vi "Lesson3 - Implicit Property Node demo.vi"() -> ()   [LabVIEW 2013]
panel:
  in  "Stop Button 2":bool
  out "Tank 2":dbl(slide) scale=0.0..10.0
  in  "Vertical Fill Slide 2":dbl(slide) scale=0.0..10.0
  in  "Vertical Fill Slide":dbl(slide) scale=0.0..10.0
  out "Tank":dbl(slide) scale=0.0..10.0
  in  "Stop Button":bool
  # "this is Property Node demonstration"
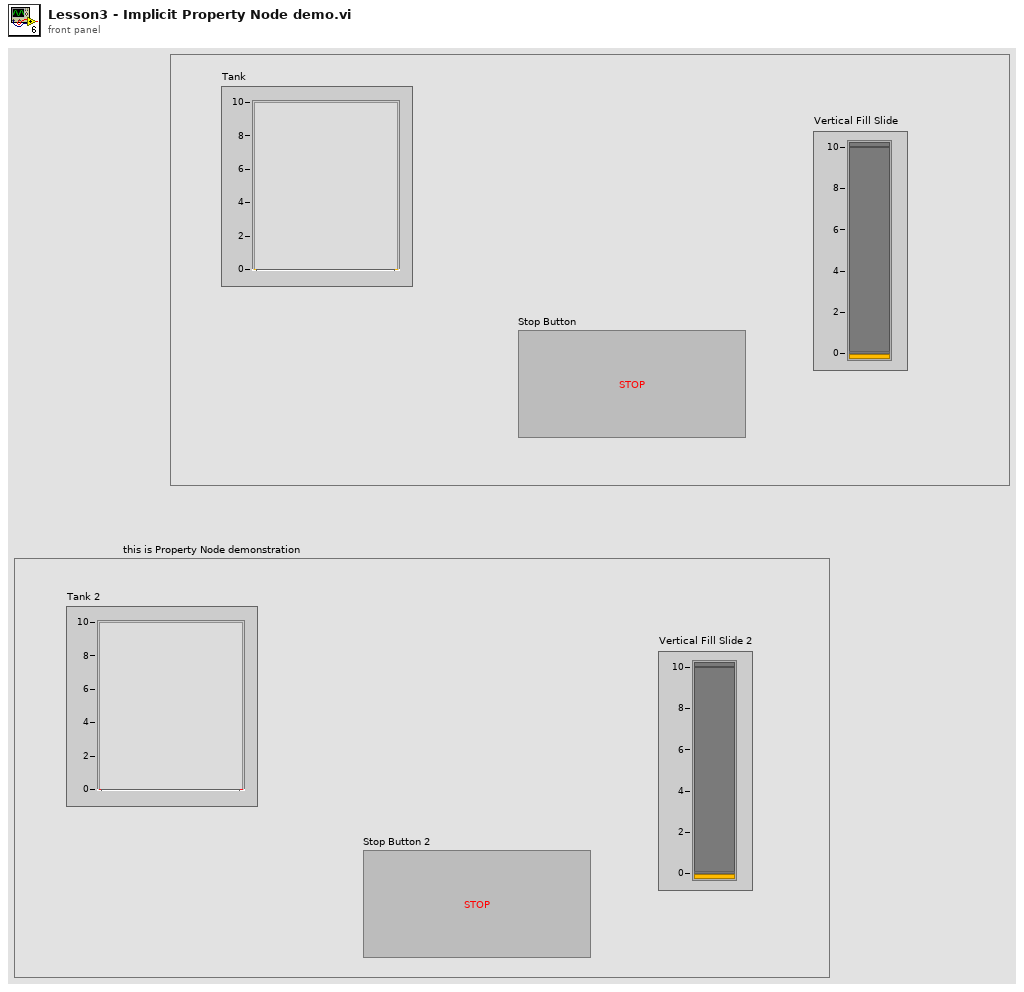
[diagram p1: front panel]
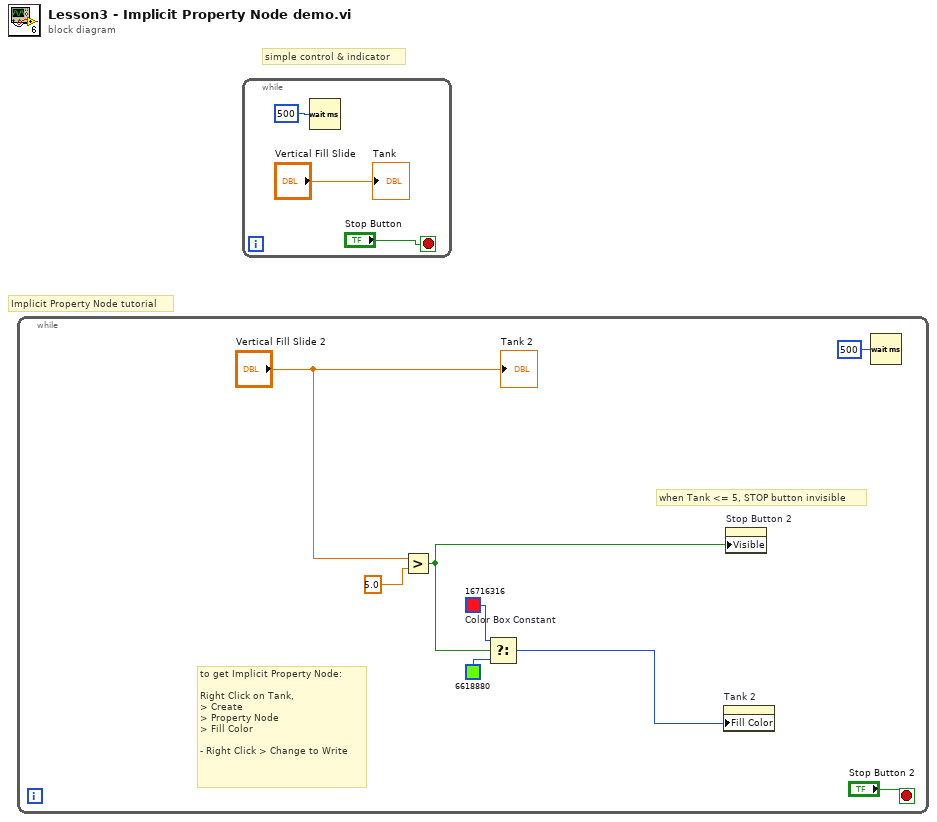
[diagram p0: block diagram]
diagram:
  # "simple control & indicator"
  # "Implicit Property Node tutorial"
  n1 = while {
    stop <- "Stop Button 2" stop-if-true
    w4 = u32 16716316  # Color Box Constant
    # "when Tank <= 5, STOP button invisible"
    # "to get Implicit Property Node:\n\nRight Click on Tank,\n> Create\n> Property Node\n> Fill Color\n\n- Right Click > Change to Write"
    n2 = Greater?(x="Vertical Fill Slide 2", y=5.0) -> (0:w1:bool)
    n3 = Select(t=w4, s=w1, f=u32 6618880) -> (s? t:f=w2:u32)
    n4 = property on="Tank 2" class="Slide (strict)"("Fill Color"=w2) -> ()  [unwired: 2 in, 2 out]
    n5 = property on="Stop Button 2" class="Bool"("Visible"=w1) -> ()  [unwired: 2 in, 2 out]
    n6 = Wait (ms)(milliseconds to wait=u32 500) -> ()  [unwired: 1 out]
    "Tank 2" <- "Vertical Fill Slide 2"
  }
  n7 = while {
    stop <- "Stop Button" stop-if-true
    n8 = Wait (ms)(milliseconds to wait=u32 500) -> ()  [unwired: 1 out]
    "Tank" <- "Vertical Fill Slide"
  }
